vi "mobileye_paser.vi"() -> ()   [LabVIEW 2015]
uses:
  G_LCM.vi
  G_mobileye_Temp.vi
panel:
  out "mobileye time":u32=2087256306
  out "XY Graph":cluster{"Y":dbl[], "Y":dbl[]}[](graph)=[{"Y"=[1.82421875, 1.8301353427767753, 1.835194070339203, 1.8394013252854347, 1.8427635002136231, 1.84528698772192, 1.8469781804084777, 1.8478434708714486, 1.8478892517089844, 1.8471219155192375, 1.84554785490036, 1.8431734624505043, 1.8400051307678222, 1.8360492524504661, 1.8313122200965881, 1.8258004263043404, 1.819520263671875, 1.8124781247973443, 1.8046804022789003, 1.796133488714695, 1.7868437767028809, 1.77681765884161, 1.7660615277290344, 1.7545817759633064, 1.742384796142578, 1.7294769808650017, 1.7158647227287291, 1.701554414331913, 1.686552448272705, 1.6708652171492577, 1.654499113559723, 1.637460530102253, 1.619755859375, 1.6013914939761162, 1.5823738265037537, 1.5627092495560646, 1.5424041557312012, 1.5214649376273155, 1.4998979878425598, 1.4777096989750862, 1.4549064636230469, 1.431494674384594, 1.4074807238578795, 1.3828710046410562, 1.3576719093322753, 1.3318898305296898, 1.3055311608314515, 1.2786022928357124, 1.251109619140625, 1.2230595323443412], "Y"=[0.0, 0.5, 1.0, 1.5, 2.0, 2.5, 3.0, 3.5, 4.0, 4.5, 5.0, 5.5, 6.0, 6.5, 7.0, 7.5, 8.0, 8.5, 9.0, 9.5, 10.0, 10.5, 11.0, 11.5, 12.0, 12.5, 13.0, 13.5, 14.0, 14.5, 15.0, 15.5, 16.0, 16.5, 17.0, 17.5, 18.0, 18.5, 19.0, 19.5, 20.0, 20.5, 21.0, 21.5, 22.0, 22.5, 23.0, 23.5, 24.0, 24.5]}, {"Y"=[-1.22265625, -1.2167396572232247, -1.211680929660797, -1.2074736747145653, -1.2041114997863769, -1.20158801227808, -1.1998968195915223, -1.1990315291285514, -1.1989857482910156, -1.1997530844807625, -1.20132714509964, -1.2037015375494957, -1.2068698692321778, -1.2108257475495339, -1.2155627799034119, -1.2210745736956596, -1.227354736328125, -1.2343968752026557, -1.2421945977210997, -1.250741511285305, -1.2600312232971191, -1.27005734115839, -1.2808134722709656, -1.2922932240366936, -1.304490203857422, -1.3173980191349983, -1.3310102772712709, -1.345320585668087, -1.360322551727295, -1.3760097828507423, -1.392375886440277, -1.409414469897747, -1.427119140625, -1.4454835060238838, -1.4645011734962463, -1.4841657504439354, -1.5044708442687988, -1.5254100623726845, -1.5469770121574402, -1.5691653010249138, -1.5919685363769531, -1.615380325615406, -1.6393942761421205, -1.6640039953589438, -1.6892030906677247, -1.7149851694703102, -1.7413438391685485, -1.7682727071642876, -1.795765380859375, -1.8238154676556588, -1.8524165749549866, -1.8815623101592065, -1.911246280670166, -1.9414620938897134, -1.972203357219696, -2.003463678061962, -2.0352366638183597, -2.0675159218907355, -2.1002950596809384, -2.1335676845908162, -2.167327404022217, -2.2015678253769875, -2.2362825560569766, -2.2714652034640315, -2.307109375, -2.3432086780667305, -2.3797567200660703, -2.4167471083998677, -2.4541734504699706, -2.4920293536782263, -2.530308425426483, -2.5690042731165885, -2.6081105041503907, -2.647620725929737, -2.687528545856476, -2.7278275713324547, -2.7685114097595216, -2.809573668539524, -2.8510079550743104, -2.892807876765728, -2.934967041015625, -2.977479055225849, -3.020337526798248, -3.0635360631346704, -3.107068271636963, -3.150927759706974, -3.1951081347465515, -3.2396030041575434, -3.284405975341797, -3.3295106557011604, -3.3749106526374817, -3.4205995735526087, -3.466571025848389, -3.51281861692667, -3.5593359541893004], "Y"=[0.0, 0.5, 1.0, 1.5, 2.0, 2.5, 3.0, 3.5, 4.0, 4.5, 5.0, 5.5, 6.0, 6.5, 7.0, 7.5, 8.0, 8.5, 9.0, 9.5, 10.0, 10.5, 11.0, 11.5, 12.0, 12.5, 13.0, 13.5, 14.0, 14.5, 15.0, 15.5, 16.0, 16.5, 17.0, 17.5, 18.0, 18.5, 19.0, 19.5, 20.0, 20.5, 21.0, 21.5, 22.0, 22.5, 23.0, 23.5, 24.0, 24.5, 25.0, 25.5, 26.0, 26.5, 27.0, 27.5, 28.0, 28.5, 29.0, 29.5, 30.0, 30.5, 31.0, 31.5, 32.0, 32.5, 33.0, 33.5, 34.0, 34.5, 35.0, 35.5, 36.0, 36.5, 37.0, 37.5, 38.0, 38.5, 39.0, 39.5, 40.0, 40.5, 41.0, 41.5, 42.0, 42.5, 43.0, 43.5, 44.0, 44.5, 45.0, 45.5, 46.0, 46.5, 47.0]}, {"Y"=[-0.94, 0.94, 0.94, -0.94, -0.94], "Y"=[-3.2, -3.2, 1.5, 1.5, -3.2]}, {"Y"=[1.984375, 1.978057861328125, 1.9718017578125, 1.965606689453125, 1.95947265625], "Y"=[0.0, 0.5, 1.0, 1.5, 2.0]}, {"Y"=[-5.28125, -5.267578125, -5.25390625, -5.240234375, -5.2265625], "Y"=[0.0, 0.5, 1.0, 1.5, 2.0]}]
  out "x_view":dbl[](array[numeric])=[0.0, 0.5, 1.0, 1.5, 2.0, 2.5, 3.0, 3.5, 4.0, 4.5, 5.0, 5.5, 6.0, 6.5, 7.0, 7.5, 8.0, 8.5, 9.0, 9.5, 10.0, 10.5, 11.0, 11.5, 12.0, 12.5, 13.0, 13.5, 14.0, 14.5, 15.0, 15.5, 16.0, 16.5, 17.0, 17.5, 18.0, 18.5, 19.0, 19.5, 20.0, 20.5, 21.0, 21.5, 22.0, 22.5, 23.0, 23.5, 24.0, 24.5, 25.0, 25.5, 26.0, 26.5, 27.0, 27.5, 28.0, 28.5, 29.0, 29.5, 30.0, 30.5, 31.0, 31.5, 32.0, 32.5, 33.0, 33.5, 34.0, 34.5, 35.0, 35.5, 36.0, 36.5, 37.0, 37.5, 38.0, 38.5, 39.0, 39.5, 40.0, 40.5, 41.0, 41.5, 42.0, 42.5, 43.0, 43.5, 44.0, 44.5, 45.0, 45.5, 46.0, 46.5, 47.0, 47.5, 48.0, 48.5, 49.0, 49.5, 50.0, 50.5, 51.0, 51.5, 52.0, 52.5, 53.0, 53.5, 54.0, 54.5, 55.0, 55.5, 56.0, 56.5, 57.0, 57.5, 58.0, 58.5, 59.0, 59.5, 60.0, 60.5, 61.0, 61.5, 62.0, 62.5, 63.0, 63.5, 64.0, 64.5, 65.0, 65.5, 66.0, 66.5, 67.0, 67.5, 68.0, 68.5, 69.0, 69.5, 70.0, 70.5, 71.0, 71.5, 72.0, 72.5, 73.0, 73.5, 74.0, 74.5, 75.0, 75.5, 76.0, 76.5, 77.0, 77.5, 78.0, 78.5, 79.0, 79.5, 80.0, 80.5, 81.0, 81.5, 82.0, 82.5, 83.0, 83.5, 84.0, 84.5, 85.0, 85.5, 86.0, 86.5, 87.0, 87.5, 88.0, 88.5, 89.0, 89.5, 90.0, 90.5, 91.0, 91.5, 92.0, 92.5, 93.0, 93.5, 94.0, 94.5, 95.0, 95.5, 96.0, 96.5, 97.0, 97.5, 98.0, 98.5, 99.0, 99.5, 100.0, 100.5, 101.0, 101.5, 102.0, 102.5, 103.0, 103.5, 104.0, 104.5, 105.0, 105.5, 106.0, 106.5, 107.0, 107.5, 108.0, 108.5, 109.0, 109.5, 110.0, 110.5, 111.0, 111.5, 112.0, 112.5, 113.0, 113.5, 114.0, 114.5, 115.0, 115.5, 116.0, 116.5, 117.0, 117.5, 118.0, 118.5, 119.0, 119.5, 120.0, 120.5, 121.0, 121.5, 122.0, 122.5, 123.0, 123.5, 124.0, 124.5, 125.0, 125.5, 126.0, 126.5, 127.0, 127.5, 128.0]
  out "M_STOP":bool
  out "M_vel_limit":dbl=70.0
  out "M_headway":dbl=inf
  out "next lane right":dbl[][](array[numeric])=[[2087253162.0, 2.0, 0.0, 3.0, 0.17, 1.984375, 0.0001220703125, 0.0, 2087254803.0, -0.0126953125, 0.0], [0.0, 0.0, 0.0, 0.0, 0.0, 0.0, 0.0, 0.0, 0.0, 0.0, 0.0], [0.0, 0.0, 0.0, 0.0, 0.0, 0.0, 0.0, 0.0, 0.0, 0.0, 0.0], [0.0, 0.0, 0.0, 0.0, 0.0, 0.0, 0.0, 0.0, 0.0, 0.0, 0.0]]
  out "next lane left":dbl[][](array[numeric])=[[2087249118.0, 2.0, 0.0, 3.0, 0.19, -5.28125, 0.0, 0.0, 2087250819.0, 0.02734375, 0.0], [0.0, 0.0, 0.0, 0.0, 0.0, 0.0, 0.0, 0.0, 0.0, 0.0, 0.0], [0.0, 0.0, 0.0, 0.0, 0.0, 0.0, 0.0, 0.0, 0.0, 0.0, 0.0], [0.0, 0.0, 0.0, 0.0, 0.0, 0.0, 0.0, 0.0, 0.0, 0.0, 0.0]]
  out "lane_right":dbl[](array[numeric])=[2087240169.0, 0.0, 2.0, 3.0, 0.18, 1.82421875, -0.001728515625, 8.52346420288086e-06, 2087241810.0, 0.0126953125, 25.046875]
  out "lane_left":dbl[](array[numeric])=[2087236146.0, 4.0, 2.0, 3.0, 0.18, -1.22265625, -0.001728515625, 8.52346420288086e-06, 2087237829.0, 0.0126953125, 47.96875]
  out "obs_tmp":dbl[][](array[numeric])=[[7.0, 29.0625, -3.75, 3.5625, 0.0, 3.0, 1.0, 0.0, 31.5, 1.55, 115.0, 2.0, 1.0, 125.59, -0.017, 5.64, 7.390000000000001, 362446576.0], [0.0, 0.0, 0.0, 0.0, 0.0, 0.0, 0.0, 0.0, 0.0, 0.0, 0.0, 0.0, 0.0, 0.0, 0.0, 0.0, 0.0, 0.0], [0.0, 0.0, 0.0, 0.0, 0.0, 0.0, 0.0, 0.0, 0.0, 0.0, 0.0, 0.0, 0.0, 0.0, 0.0, 0.0, 0.0, 0.0], [0.0, 0.0, 0.0, 0.0, 0.0, 0.0, 0.0, 0.0, 0.0, 0.0, 0.0, 0.0, 0.0, 0.0, 0.0, 0.0, 0.0, 0.0], [0.0, 0.0, 0.0, 0.0, 0.0, 0.0, 0.0, 0.0, 0.0, 0.0, 0.0, 0.0, 0.0, 0.0, 0.0, 0.0, 0.0, 0.0], [0.0, 0.0, 0.0, 0.0, 0.0, 0.0, 0.0, 0.0, 0.0, 0.0, 0.0, 0.0, 0.0, 0.0, 0.0, 0.0, 0.0, 0.0], [0.0, 0.0, 0.0, 0.0, 0.0, 0.0, 0.0, 0.0, 0.0, 0.0, 0.0, 0.0, 0.0, 0.0, 0.0, 0.0, 0.0, 0.0], [0.0, 0.0, 0.0, 0.0, 0.0, 0.0, 0.0, 0.0, 0.0, 0.0, 0.0, 0.0, 0.0, 0.0, 0.0, 0.0, 0.0, 0.0], [0.0, 0.0, 0.0, 0.0, 0.0, 0.0, 0.0, 0.0, 0.0, 0.0, 0.0, 0.0, 0.0, 0.0, 0.0, 0.0, 0.0, 0.0], [0.0, 0.0, 0.0, 0.0, 0.0, 0.0, 0.0, 0.0, 0.0, 0.0, 0.0, 0.0, 0.0, 0.0, 0.0, 0.0, 0.0, 0.0], [0.0, 0.0, 0.0, 0.0, 0.0, 0.0, 0.0, 0.0, 0.0, 0.0, 0.0, 0.0, 0.0, 0.0, 0.0, 0.0, 0.0, 0.0], [0.0, 0.0, 0.0, 0.0, 0.0, 0.0, 0.0, 0.0, 0.0, 0.0, 0.0, 0.0, 0.0, 0.0, 0.0, 0.0, 0.0, 0.0], [0.0, 0.0, 0.0, 0.0, 0.0, 0.0, 0.0, 0.0, 0.0, 0.0, 0.0, 0.0, 0.0, 0.0, 0.0, 0.0, 0.0, 0.0], [0.0, 74.9375, 0.0, 0.0, 0.0, 0.0, 0.0, 0.0, 0.0, 0.0, 0.0, 0.0, 0.0, 0.0, 0.0, 0.0, 0.0, 0.0], [0.0, 0.0, 0.0, 0.0, 0.0, 0.0, 0.0, 0.0, 0.0, 0.0, 0.0, 0.0, 0.0, 0.0, 0.0, 0.0, 0.0, 0.0], [0.0, 0.0, 0.0, 0.0, 0.0, 0.0, 0.0, 0.0, 0.0, 0.0, 0.0, 0.0, 0.0, 0.0, 0.0, 0.0, 0.0, 0.0], [0.0, 0.0, 0.0, 0.0, 0.0, 0.0, 0.0, 0.0, 0.0, 0.0, 0.0, 0.0, 0.0, 0.0, 0.0, 0.0, 0.0, 0.0], [0.0, 0.0, 0.0, 0.0, 0.0, 0.0, 0.0, 0.0, 0.0, 0.0, 0.0, 0.0, 0.0, 0.0, 0.0, 0.0, 0.0, 0.0], [0.0, 0.0, 0.0, 0.0, 0.0, 0.0, 0.0, 0.0, 0.0, 0.0, 0.0, 0.0, 0.0, 0.0, 0.0, 0.0, 0.0, 0.0], [0.0, 0.0, 0.0, 0.0, 0.0, 0.0, 0.0, 0.0, 0.0, 0.0, 0.0, 0.0, 0.0, 0.0, 0.0, 0.0, 0.0, 0.0], [0.0, 0.0, 0.0, 0.0, 0.0, 0.0, 0.0, 0.0, 0.0, 0.0, 0.0, 0.0, 0.0, 0.0, 0.0, 0.0, 0.0, 0.0], [0.0, 0.0, 0.0, 0.0, 0.0, 0.0, 0.0, 0.0, 0.0, 0.0, 0.0, 0.0, 0.0, 0.0, 0.0, 0.0, 0.0, 0.0], [0.0, 0.0, 0.0, 0.0, 0.0, 0.0, 0.0, 0.0, 0.0, 0.0, 0.0, 0.0, 0.0, 0.0, 0.0, 0.0, 0.0, 0.0], [0.0, 0.0, 0.0, 0.0, 0.0, 0.0, 0.0, 0.0, 0.0, 0.0, 0.0, 0.0, 0.0, 0.0, 0.0, 0.0, 0.0, 0.0], [0.0, 0.0, 0.0, 0.0, 0.0, 0.0, 0.0, 0.0, 0.0, 0.0, 0.0, 0.0, 0.0, 0.0, 0.0, 0.0, 0.0, 0.0], [0.0, 0.0, 0.0, 0.0, 0.0, 0.0, 0.0, 0.0, 0.0, 0.0, 0.0, 0.0, 0.0, 0.0, 0.0, 0.0, 0.0, 0.0], [0.0, 0.0, 0.0, 0.0, 0.0, 0.0, 0.0, 0.0, 0.0, 0.0, 0.0, 0.0, 0.0, 0.0, 0.0, 0.0, 0.0, 0.0], [0.0, 0.0, 0.0, 0.0, 0.0, 0.0, 0.0, 0.0, 0.0, 0.0, 0.0, 0.0, 0.0, 0.0, 0.0, 0.0, 0.0, 0.0], [0.0, 0.0, 0.0, 0.0, 0.0, 0.0, 0.0, 0.0, 0.0, 0.0, 0.0, 0.0, 0.0, 0.0, 0.0, 0.0, 0.0, 0.0], [0.0, 0.0, 0.0, 0.0, 0.0, 0.0, 0.0, 0.0, 0.0, 0.0, 0.0, 0.0, 0.0, 0.0, 0.0, 0.0, 0.0, 0.0], [0.0, 0.0, 0.0, 0.0, 0.0, 0.0, 0.0, 0.0, 0.0, 0.0, 0.0, 0.0, 0.0, 0.0, 0.0, 0.0, 0.0, 0.0], [0.0, 0.0, 0.0, 0.0, 0.0, 0.0, 0.0, 0.0, 0.0, 0.0, 0.0, 0.0, 0.0, 0.0, 0.0, 0.0, 0.0, 0.0], [0.0, 0.0, 0.0, 0.0, 0.0, 0.0, 0.0, 0.0, 0.0, 0.0, 0.0, 0.0, 0.0, 0.0, 0.0, 0.0, 0.0, 0.0], [0.0, 0.0, 0.0, 0.0, 0.0, 0.0, 0.0, 0.0, 0.0, 0.0, 0.0, 0.0, 0.0, 0.0, 0.0, 0.0, 0.0, 0.0], [0.0, 0.0, 0.0, 0.0, 0.0, 0.0, 0.0, 0.0, 0.0, 0.0, 0.0, 0.0, 0.0, 0.0, 0.0, 0.0, 0.0, 0.0], [0.0, 0.0, 0.0, 0.0, 0.0, 0.0, 0.0, 0.0, 0.0, 0.0, 0.0, 0.0, 0.0, 0.0, 0.0, 0.0, 0.0, 0.0], [0.0, 0.0, 0.0, 0.0, 0.0, 0.0, 0.0, 0.0, 0.0, 0.0, 0.0, 0.0, 0.0, 0.0, 0.0, 0.0, 0.0, 0.0], [0.0, 0.0, 0.0, 0.0, 0.0, 0.0, 0.0, 0.0, 0.0, 0.0, 0.0, 0.0, 0.0, 0.0, 0.0, 0.0, 0.0, 0.0], [0.0, 0.0, 0.0, 0.0, 0.0, 0.0, 0.0, 0.0, 0.0, 0.0, 0.0, 0.0, 0.0, 0.0, 0.0, 0.0, 0.0, 0.0], [0.0, 0.0, 0.0, 0.0, 0.0, 0.0, 0.0, 0.0, 0.0, 0.0, 0.0, 0.0, 0.0, 0.0, 0.0, 0.0, 0.0, 0.0], [0.0, 0.0, 0.0, 0.0, 0.0, 0.0, 0.0, 0.0, 0.0, 0.0, 0.0, 0.0, 0.0, 0.0, 0.0, 0.0, 0.0, 0.0], [0.0, 0.0, 0.0, 0.0, 0.0, 0.0, 0.0, 0.0, 0.0, 0.0, 0.0, 0.0, 0.0, 0.0, 0.0, 0.0, 0.0, 0.0], [0.0, 0.0, 0.0, 0.0, 0.0, 0.0, 0.0, 0.0, 0.0, 0.0, 0.0, 0.0, 0.0, 0.0, 0.0, 0.0, 0.0, 0.0], [0.0, 0.0, 0.0, 0.0, 0.0, 0.0, 0.0, 0.0, 0.0, 0.0, 0.0, 0.0, 0.0, 0.0, 0.0, 0.0, 0.0, 0.0], [0.0, 0.0, 0.0, 0.0, 0.0, 0.0, 0.0, 0.0, 0.0, 0.0, 0.0, 0.0, 0.0, 0.0, 0.0, 0.0, 0.0, 0.0], [0.0, 0.0, 0.0, 0.0, 0.0, 0.0, 0.0, 0.0, 0.0, 0.0, 0.0, 0.0, 0.0, 0.0, 0.0, 0.0, 0.0, 0.0], [0.0, 0.0, 0.0, 0.0, 0.0, 0.0, 0.0, 0.0, 0.0, 0.0, 0.0, 0.0, 0.0, 0.0, 0.0, 0.0, 0.0, 0.0], [0.0, 0.0, 0.0, 0.0, 0.0, 0.0, 0.0, 0.0, 0.0, 0.0, 0.0, 0.0, 0.0, 0.0, 0.0, 0.0, 0.0, 0.0], [0.0, 0.0, 0.0, 0.0, 0.0, 0.0, 0.0, 0.0, 0.0, 0.0, 0.0, 0.0, 0.0, 0.0, 0.0, 0.0, 0.0, 0.0], [0.0, 0.0, 0.0, 0.0, 0.0, 0.0, 0.0, 0.0, 0.0, 0.0, 0.0, 0.0, 0.0, 0.0, 0.0, 0.0, 0.0, 0.0], [0.0, 0.0, 0.0, 0.0, 0.0, 0.0, 0.0, 0.0, 0.0, 0.0, 0.0, 0.0, 0.0, 0.0, 0.0, 0.0, 0.0, 0.0], [0.0, 0.0, 0.0, 0.0, 0.0, 0.0, 0.0, 0.0, 0.0, 0.0, 0.0, 0.0, 0.0, 0.0, 0.0, 0.0, 0.0, 0.0], [0.0, 0.0, 0.0, 0.0, 0.0, 0.0, 0.0, 0.0, 0.0, 0.0, 0.0, 0.0, 0.0, 0.0, 0.0, 0.0, 0.0, 0.0], [0.0, 0.0, 0.0, 0.0, 0.0, 0.0, 0.0, 0.0, 0.0, 0.0, 0.0, 0.0, 0.0, 0.0, 0.0, 0.0, 0.0, 0.0], [0.0, 0.0, 0.0, 0.0, 0.0, 0.0, 0.0, 0.0, 0.0, 0.0, 0.0, 0.0, 0.0, 0.0, 0.0, 0.0, 0.0, 0.0], [0.0, 0.0, 0.0, 0.0, 0.0, 0.0, 0.0, 0.0, 0.0, 0.0, 0.0, 0.0, 0.0, 0.0, 0.0, 0.0, 0.0, 0.0], [0.0, 0.0, 0.0, 0.0, 0.0, 0.0, 0.0, 0.0, 0.0, 0.0, 0.0, 0.0, 0.0, 0.0, 0.0, 0.0, 0.0, 0.0], [0.0, 0.0, 0.0, 0.0, 0.0, 0.0, 0.0, 0.0, 0.0, 0.0, 0.0, 0.0, 0.0, 0.0, 0.0, 0.0, 0.0, 0.0], [0.0, 0.0, 0.0, 0.0, 0.0, 0.0, 0.0, 0.0, 0.0, 0.0, 0.0, 0.0, 0.0, 0.0, 0.0, 0.0, 0.0, 0.0], [0.0, 0.0, 0.0, 0.0, 0.0, 0.0, 0.0, 0.0, 0.0, 0.0, 0.0, 0.0, 0.0, 0.0, 0.0, 0.0, 0.0, 0.0], [0.0, 0.0, 0.0, 0.0, 0.0, 0.0, 0.0, 0.0, 0.0, 0.0, 0.0, 0.0, 0.0, 0.0, 0.0, 0.0, 0.0, 0.0], [0.0, 0.0, 0.0, 0.0, 0.0, 0.0, 0.0, 0.0, 0.0, 0.0, 0.0, 0.0, 0.0, 0.0, 0.0, 0.0, 0.0, 0.0], [0.0, 0.0, 0.0, 0.0, 0.0, 0.0, 0.0, 0.0, 0.0, 0.0, 0.0, 0.0, 0.0, 0.0, 0.0, 0.0, 0.0, 0.0], [0.0, 0.0, 0.0, 0.0, 0.0, 0.0, 0.0, 0.0, 0.0, 0.0, 0.0, 0.0, 0.0, 0.0, 0.0, 0.0, 0.0, 0.0]]
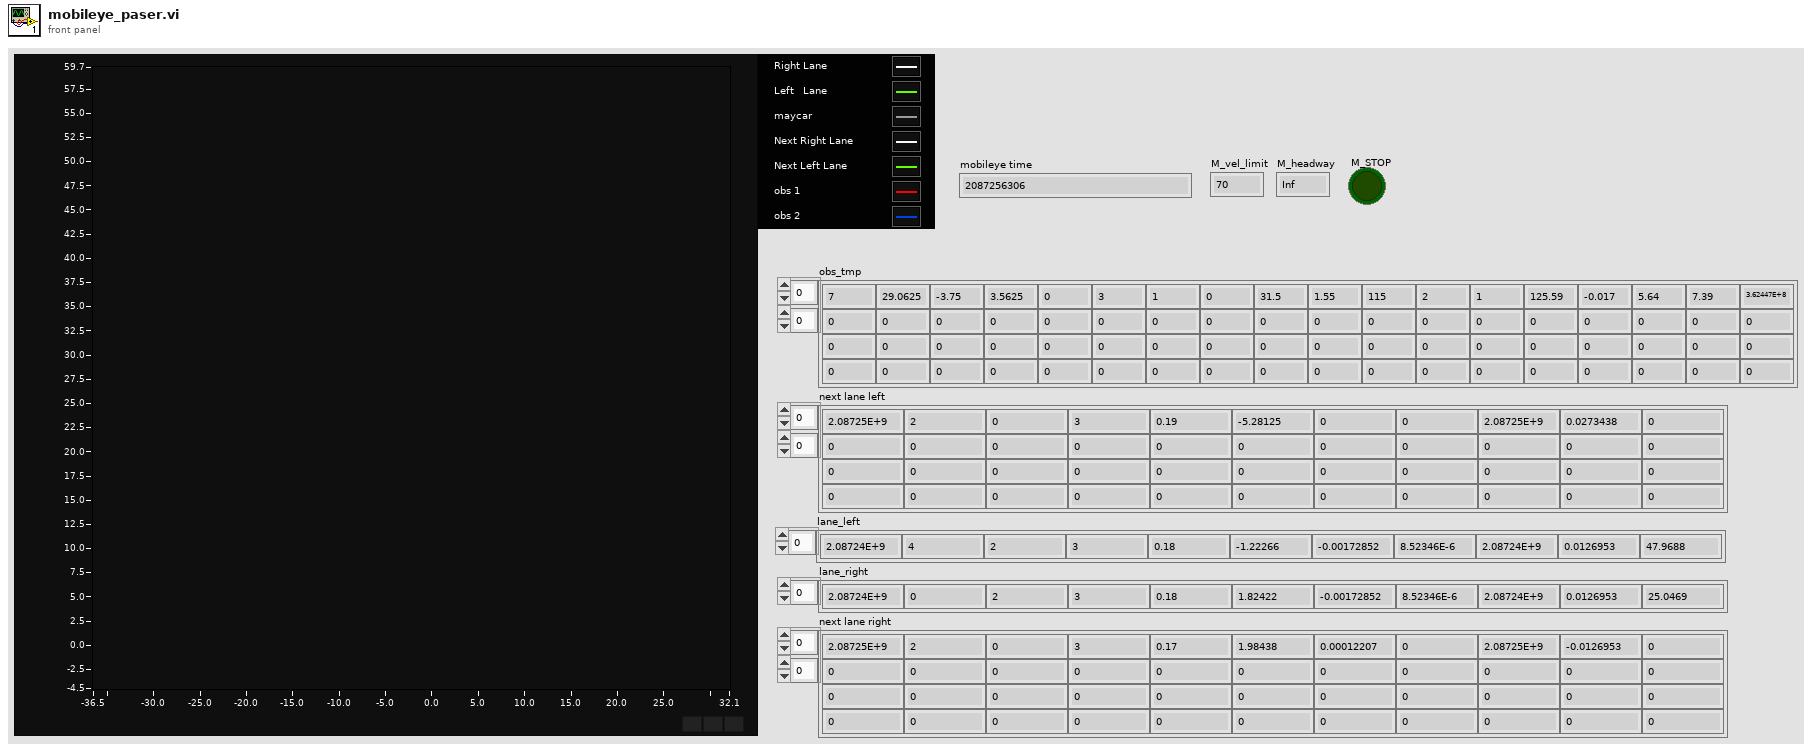
[diagram p1: front panel]
types:
  T1 = cluster{"hash":i64, "sys time":i64, "mobileye time":u32, "ID":u32, "data":u8[]}
  T2 = cluster{"identifier":u32, "timestamp":timestamp, "payload":u8[]}
  T3 = cluster{"hash":i64, "sys time":i64, "car time":u32, "ID":u32, "data":u8[]}
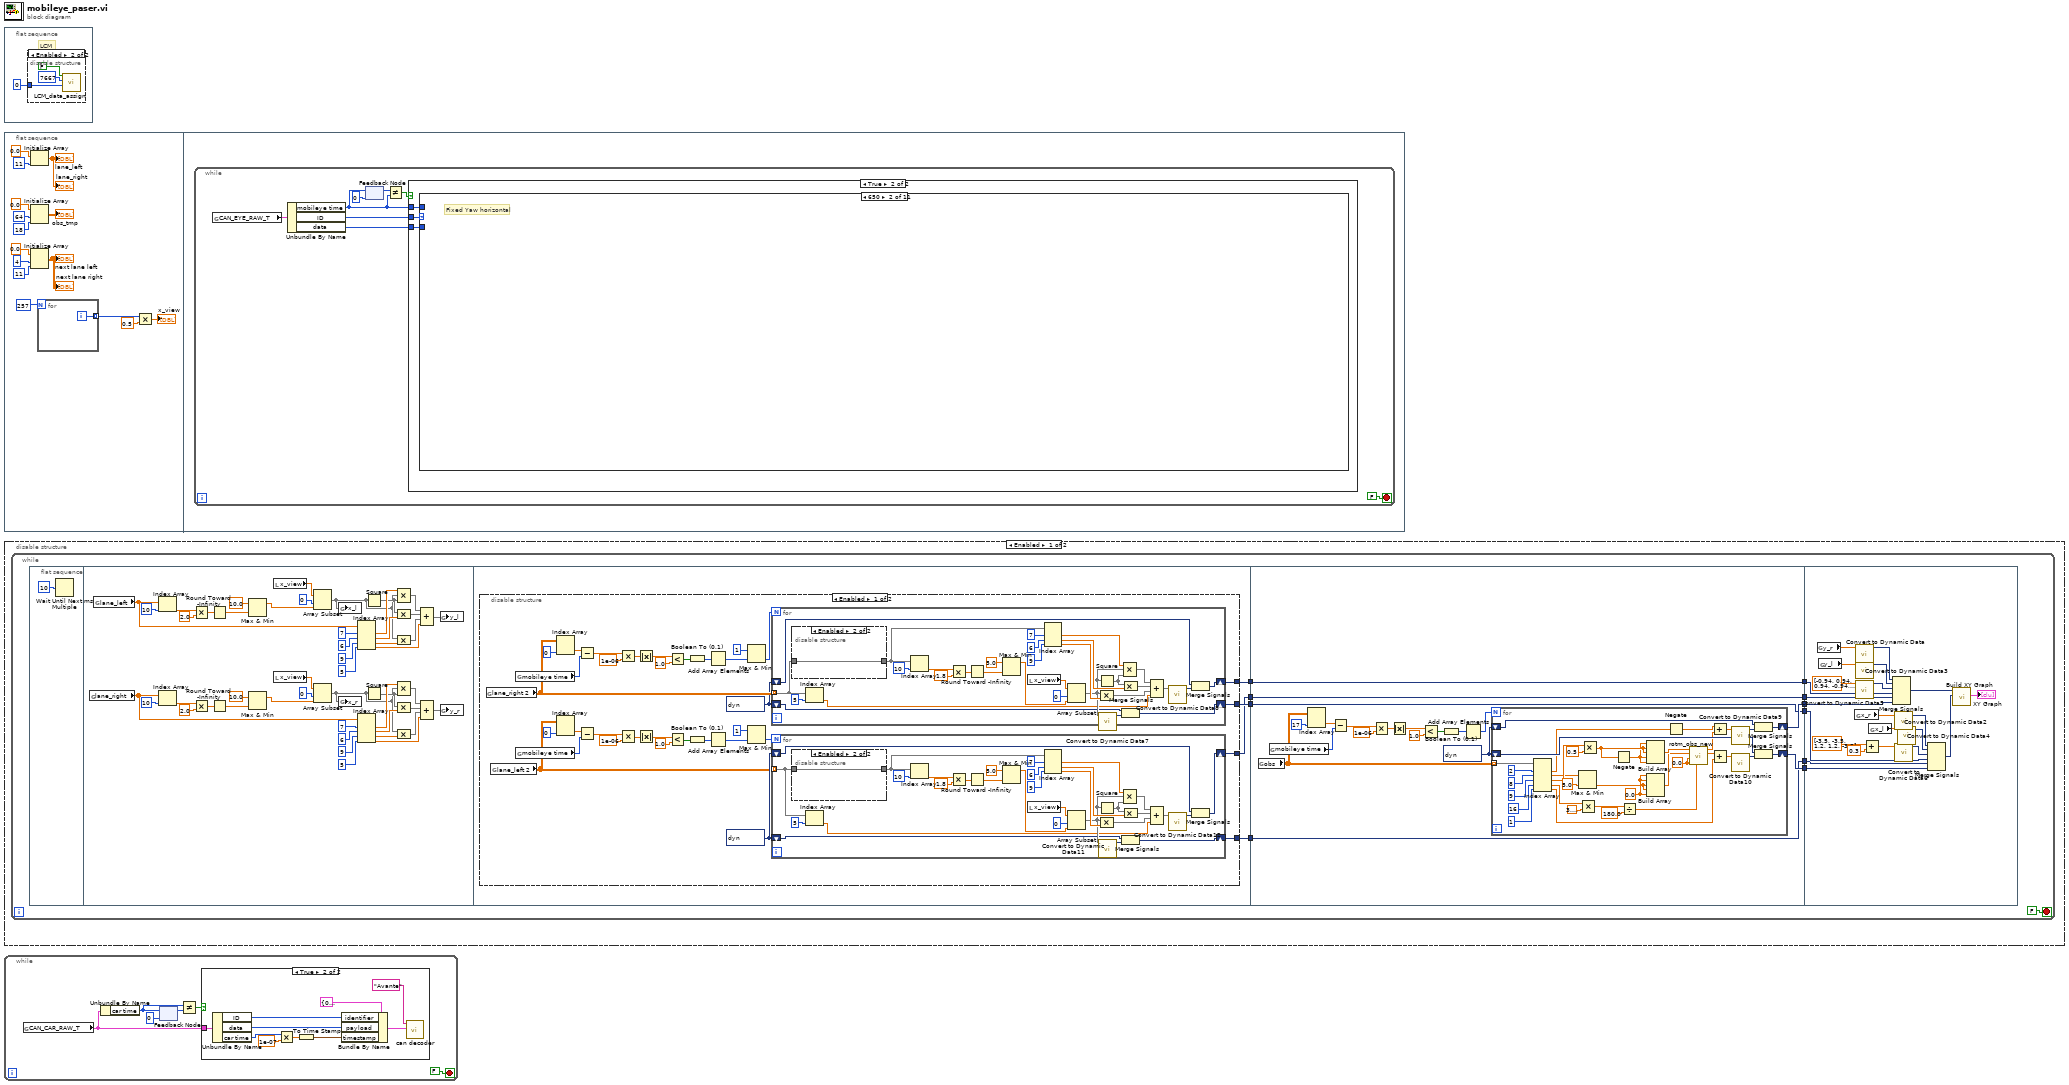
[diagram p0: block diagram]
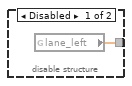
[diagram p3: hidden frame]
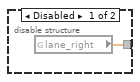
[diagram p4: hidden frame]
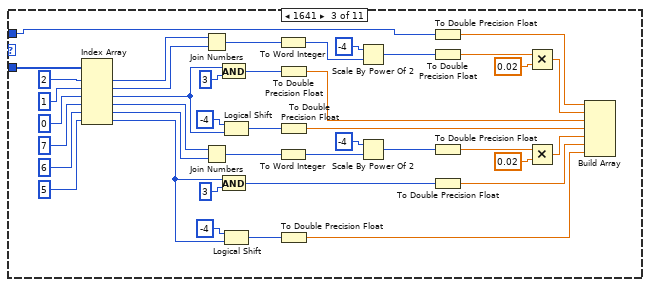
[diagram p9: hidden frame]
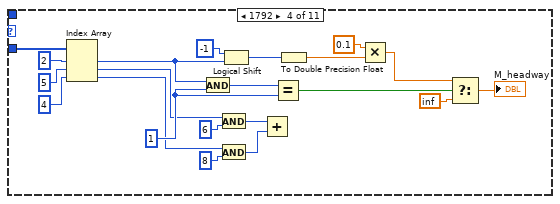
[diagram p10: hidden frame]
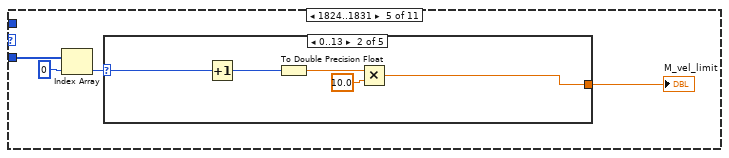
[diagram p11: hidden frame]
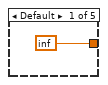
[diagram p12: hidden frame]
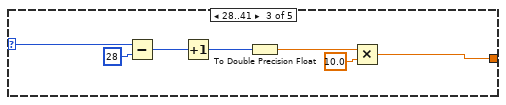
[diagram p13: hidden frame]
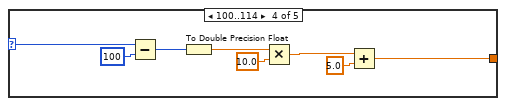
[diagram p14: hidden frame]
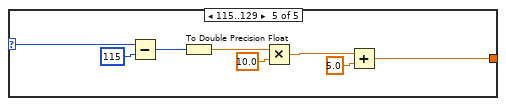
[diagram p15: hidden frame]
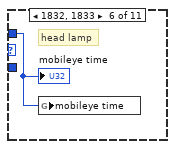
[diagram p16: hidden frame]
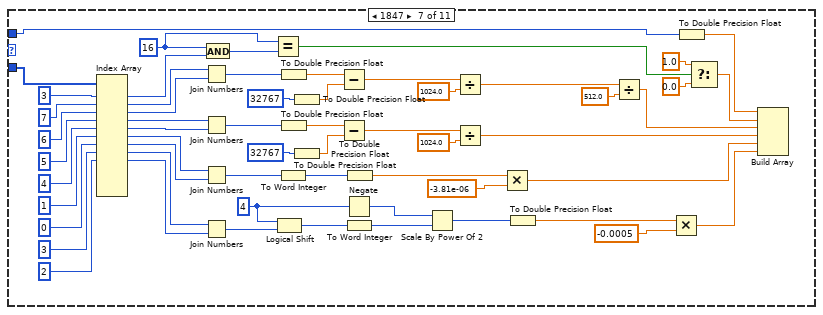
[diagram p17: hidden frame]
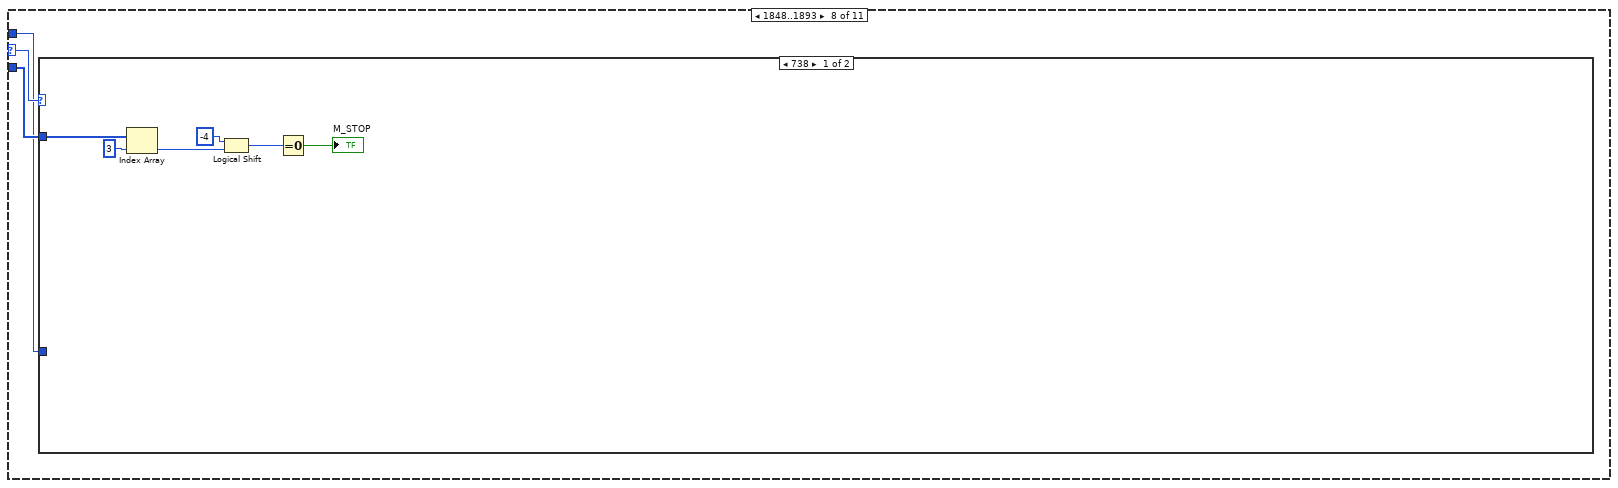
[diagram p18: hidden frame]
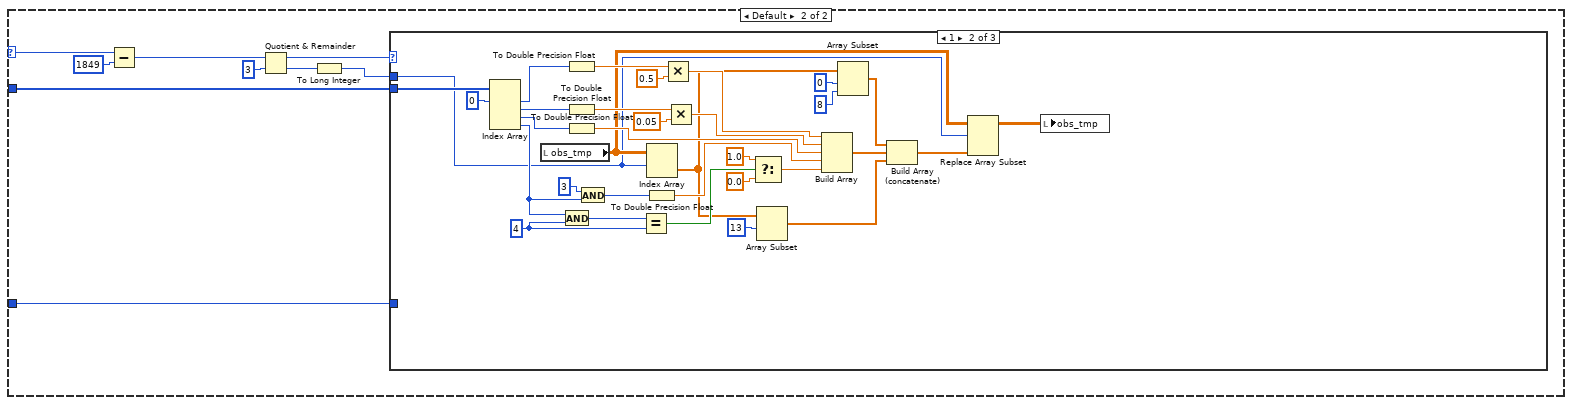
[diagram p19: hidden frame]
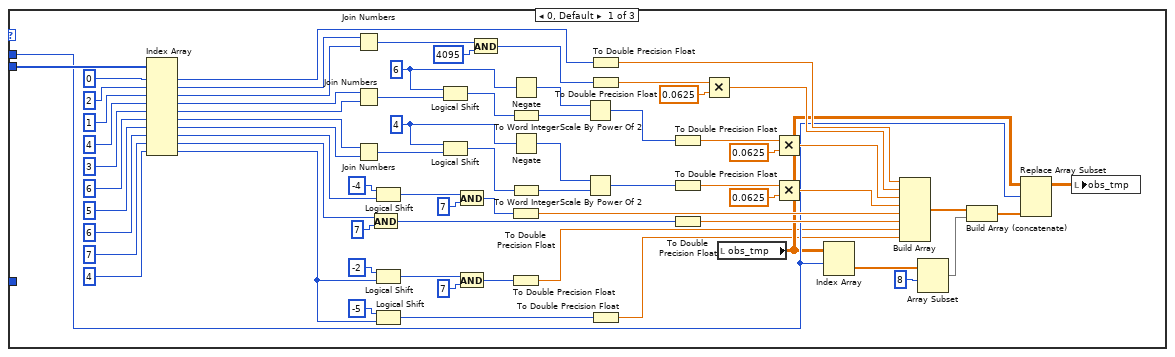
[diagram p20: hidden frame]
diagram:
  n1 = flat-sequence {
    frame #0 {
      # "LCM"
      n2 = disable-structure shown="Enabled" {
        disable-tunnel: u16 0 ("time-to-live") -> [_ w2]
        frame Disabled {
          n3 = call "comm.vi"() -> ()  [unwired: 12 in]
        }
        frame Enabled {
          n4 = call "LCM_data_assign.vi"("time-to-live"=w2, "port"=u16 7667, "velodyne enable"=FALSE) -> ()  [unwired: 9 in]
        }
      }
    }
  }
  n5 = flat-sequence {
    frame #0 {
      n6 = Initialize Array(0.0, 11 ("dimension size")) -> (→"lane_left" →"lane_right":dbl[])
      n7 = Initialize Array(0.0 ("element"), 64 ("dimension size"), 18 ("dimension size")) -> (→"obs_tmp":dbl[][])
      n8 = Initialize Array(0.0, 4 ("dimension size"), 11 ("dimension size")) -> (→"next lane right" →"next lane left":dbl[][])
      n9 = for {
        N: 257 -> [_]
        tunnel: [w20] -> w11 mode=indexing
        i -> [w20]
      }
      n10 = Multiply(x=w11, y=0.5) -> (x*y=→"x_view":dbl[])
    }
    frame #1 {
      n11 = while {
        stop <- FALSE stop-if-true
        n12 = global read "G_LCM.vi" "CAN_EYE_RAW_T"() -> (w27:T1)
        n13 = Unbundle By Name(w27) -> ("mobileye time"=w22:u32, "ID"=w23:u32, "data"=w24:u8[])
        n14 = feedback #1(u32 0 ("mobileye time")) -> (w21:u32)
        n15 = feedback-in #1(w22) -> ()
        n16 = Not Equal?(x=w21, y=w22) -> (x != y?=w25:bool)
        n17 = case shown="True" w25 {
          tunnel: w24 -> [_ w31]
          tunnel: w22 -> [_ w30]
          tunnel: w23 -> [_ w29]
          frame False {
          }
          frame True {
            n18 = case shown="650" w29 {
              selector: w29 -> [_ _ _ _ _ _ _ w187 _ w393 w475]
              tunnel: w31 -> [_ _ w72 w93 w97 _ w184 w186 w362 w447 w502]
              tunnel: w30 -> [_ _ w49 _ _ w127 w131 w185 _ w413 w478]
              frame 0, Default {
              }
              frame 1616 {
                # "Fixed Yaw horizontal"
              }
              frame 1641 {
                n19 = Index Array(array=w72, index #1=2 ("index"), index #2=1 ("index"), index #3=0 ("index"), index #4=7 ("index"), index #5=6 ("index"), index #6=5 ("index")) -> (element #1=w69:u8, element #2=w68:u8, element #3=w47:u8, element #4=w40:u8, element #5=w39:u8, element #6=w35:u8)
                n20 = Join Numbers(hi=w69, lo=w68) -> ((hi.lo)=w67:u16)
                n21 = Join Numbers(hi=w40, lo=w39) -> ((hi.lo)=w62:u16)
                n22 = And(x=w47, y=u8 3) -> (x .and. y?=w46:u8)
                n23 = And(x=w35, y=u8 3) -> (x .and. y?=w38:u8)
                n24 = Logical Shift(y=i16 -4, x=w47) -> (x << y=w45:u8)
                n25 = Logical Shift(y=i16 -4, x=w35) -> (x << y=w42:u8)
                n26 = To Word Integer(number=w67) -> (16bit integer=w54:i16)
                n27 = To Word Integer(number=w62) -> (16bit integer=w51:i16)
                n28 = To Double Precision Float(number=w46) -> (double precision float=w44:dbl)
                n29 = To Double Precision Float(number=w45) -> (double precision float=w43:dbl)
                n30 = To Double Precision Float(number=w42) -> (double precision float=w36:dbl)
                n31 = Scale By Power Of 2(n=i16 -4 ("y"), x=w54) -> (x*2^n=w53:i16)
                n32 = Scale By Power Of 2(n=i16 -4 ("y"), x=w51) -> (x*2^n=w50:i16)
                n33 = To Double Precision Float(number=w49) -> (double precision float=w34:dbl)
                n34 = To Double Precision Float(number=w53) -> (double precision float=w66:dbl)
                n35 = To Double Precision Float(number=w50) -> (double precision float=w63:dbl)
                n36 = To Double Precision Float(number=w38) -> (double precision float=w37:dbl)
                n37 = Multiply(x=w66, y=0.02) -> (x*y=w33:dbl)
                n38 = Multiply(x=w63, y=0.02) -> (x*y=w32:dbl)
                n39 = Build Array(w34, w33, w44, w43, w32, w37, w36) -> ()  [unwired: 1 out]
              }
              frame 1792 {
                w88 = u8 1 ("y")
                n40 = Index Array(array=w93, index #1=2 ("index"), index #2=5 ("index"), index #3=4 ("index")) -> (element #1=w91:u8, element #2=w80:u8, element #3=w76:u8)
                n41 = And(x=w91, y=w88) -> (x .and. y?=w89:u8)
                n42 = And(x=w80, y=u8 6) -> (x .and. y?=w75:u8)
                n43 = And(x=w76, y=u8 8) -> (x .and. y?=w74:u8)
                n44 = Logical Shift(y=i16 -1, x=w91) -> (x << y=w86:u8)
                n45 = Add(x=w75, y=w74) -> ()  [unwired: 1 out]
                n46 = Equal?(x=w89, y=w88) -> (x = y?=w87:bool)
                n47 = To Double Precision Float(number=w86) -> (double precision float=w85:dbl)
                n48 = Multiply(x=0.1, y=w85) -> (x*y=w83:dbl)
                n49 = Select(t=w83, s=w87, f=inf) -> (s? t:f=→"M_headway":dbl)
              }
              frame 1824..1831 {
                n50 = Index Array(array=w97, index=0) -> (element=w95:u8)
                n51 = case shown="0..13" w95 {
                  selector: w95 -> [_ w103 w106 w116 w124]
                  tunnel: [inf w99 w107 w111 w119] -> w94
                  frame Default {
                  }
                  frame 0..13 {
                    n52 = Increment(x=w103) -> (x+1=w102:u8)
                    n53 = To Double Precision Float(number=w102) -> (double precision float=w101:dbl)
                    n54 = Multiply(x=w101, y=10.0) -> (x*y=w99:dbl)
                  }
                  frame 28..41 {
                    n55 = Subtract(x=w106, y=u8 28) -> (x-y=w105:u8)
                    n56 = Increment(x=w105) -> (x+1=w110:u8)
                    n57 = To Double Precision Float(number=w110) -> (double precision float=w109:dbl)
                    n58 = Multiply(x=w109, y=10.0) -> (x*y=w107:dbl)
                  }
                  frame 100..114 {
                    n59 = Subtract(x=w116, y=u8 100) -> (x-y=w114:u8)
                    n60 = To Double Precision Float(number=w114) -> (double precision float=w118:dbl)
                    n61 = Multiply(x=w118, y=10.0) -> (x*y=w113:dbl)
                    n62 = Add(x=w113, y=5.0) -> (x+y=w111:dbl)
                  }
                  frame 115..129 {
                    n63 = Subtract(x=w124, y=u8 115) -> (x-y=w122:u8)
                    n64 = To Double Precision Float(number=w122) -> (double precision float=w126:dbl)
                    n65 = Multiply(x=w126, y=10.0) -> (x*y=w121:dbl)
                    n66 = Add(x=w121, y=5.0) -> (x+y=w119:dbl)
                  }
                }
                "M_vel_limit" <- w94
              }
              frame 1832, 1833 {
                # "head lamp"
                n67 = global write "G_mobileye_Temp.vi" "mobileye time"(w127) -> ()
                "mobileye time" <- w127
              }
              frame 1847 {
                w164 = u8 16 ("x")
                w166 = i16 4 ("x")
                n68 = Index Array(array=w184, index #1=3 ("index"), index #2=7 ("index"), index #3=6 ("index"), index #4=5 ("index"), index #5=4 ("index"), index #6=1 ("index"), index #7=0 ("index"), index #8=3 ("index"), index #9=2 ("index")) -> (element #1=w147:u8, element #2=w141:u8, element #3=w140:u8, element #4=w139:u8, element #5=w138:u8, element #6=w181:u8, element #7=w180:u8, element #8=w173:u8, element #9=w172:u8)  [unwired: 4 in, 4 out]
                n69 = Join Numbers(hi=w141, lo=w140) -> ((hi.lo)=w163:u16)
                n70 = Join Numbers(hi=w139, lo=w138) -> ((hi.lo)=w151:u16)
                n71 = Join Numbers(hi=w181, lo=w180) -> ((hi.lo)=w179:u16)
                n72 = Join Numbers(hi=w173, lo=w172) -> ((hi.lo)=w169:u16)
                n73 = And(x=w164, y=w147) -> (x .and. y?=w165:u8)
                n74 = Equal?(x=w164, y=w165) -> (x = y?=w150:bool)
                n75 = Logical Shift(y=w166, x=w169) -> (x << y=w171:u16)
                n76 = To Word Integer(number=w179) -> (16bit integer=w178:i16)
                n77 = To Double Precision Float(number=w163) -> (double precision float=w162:dbl)
                n78 = To Double Precision Float(number=w151) -> (double precision float=w152:dbl)
                n79 = To Double Precision Float(number=i16 32767) -> (double precision float=w160:dbl)
                n80 = To Double Precision Float(number=i16 32767) -> (double precision float=w154:dbl)
                n81 = Subtract(x=w162, y=w160) -> (x-y=w159:dbl)
                n82 = Subtract(x=w152, y=w154) -> (x-y=w155:dbl)
                n83 = Negate(x=w166) -> (-x=w168:i16)
                n84 = To Word Integer(number=w171) -> (16bit integer=w128:i16)
                n85 = To Double Precision Float(number=w178) -> (double precision float=w177:dbl)
                n86 = Scale By Power Of 2(n=w168, x=w128) -> (x*2^n=w167:i16)
                n87 = Divide(x=w159, y=1024.0) -> (x/y=w136:dbl)
                n88 = Divide(x=w155, y=1024.0) -> (x/y=w134:dbl)
                n89 = Multiply(x=w177, y=-3.81e-06) -> (x*y=w133:dbl)
                n90 = To Double Precision Float(number=w167) -> (double precision float=w129:dbl)
                n91 = Divide(x=w136, y=512.0) -> (x/y=w135:dbl)
                n92 = Multiply(x=w129, y=-0.0005) -> (x*y=w132:dbl)
                n93 = To Double Precision Float(number=w131) -> (double precision float=w130:dbl)
                n94 = Select(t=1.0, s=w150, f=0.0) -> (s? t:f=w137:dbl)
                n95 = Build Array(w130, w137, w135, w134, w133, w132) -> ()  [unwired: 1 out]
              }
              frame 1848..1893 {
                n96 = case shown="738" w187 {
                  selector: w187 -> [_ w196]
                  tunnel: w186 -> [w193 w198]
                  tunnel: w185 -> [_ w194]
                  frame 1848 {
                    n97 = Index Array(array=w193, index=3) -> (element=w189:u8)
                    n98 = Logical Shift(y=i16 -4, x=w189) -> (x << y=w191:u8)
                    n99 = Equal To 0?(x=w191) -> (x = 0?=→"M_STOP":bool)
                  }
                  frame Default {
                    n100 = Subtract(x=w196, y=u32 1849) -> (x-y=w201:u32)
                    n101 = Quotient & Remainder(x=w201, y=u32 3) -> (x-y*floor(x/y)=w199:u32, floor(x/y)=w197:u32)
                    n102 = To Long Integer(number=w197) -> (32bit integer=w195:i32)
                    n103 = case shown="1" w199 {
                      tunnel: w198 -> [w272 w305 w308]
                      tunnel: w195 -> [w226 w280 w307]
                      tunnel: w194 -> [_ _ w306]
                      frame 0, Default {
                        w215 = i16 4 ("y")
                        w219 = i16 6 ("y")
                        n104 = Index Array(array=w272, index #1=0 ("index"), index #2=2 ("index"), index #3=1 ("index"), index #4=4 ("index"), index #5=3 ("index"), index #6=6 ("index"), index #7=5 ("index"), index #8=6 ("index"), index #9=7 ("index"), index #10=4 ("index")) -> (element #1=w264:u8, element #2=w268:u8, element #3=w267:u8, element #4=w256:u8, element #5=w255:u8, element #6=w243:u8, element #7=w242:u8, element #8=w238:u8, element #9=w231:u8, element #10=w206:u8)
                        n105 = Join Numbers(hi=w268, lo=w267) -> ((hi.lo)=w259:u16)
                        n106 = Join Numbers(hi=w256, lo=w255) -> ((hi.lo)=w254:u16)
                        n107 = Join Numbers(hi=w243, lo=w242) -> ((hi.lo)=w244:u16)
                        n108 = And(x=w231, y=u8 7) -> (x .and. y?=w230:u8)
                        n109 = Logical Shift(y=i16 -4, x=w238) -> (x << y=w237:u8)
                        n110 = Logical Shift(y=i16 -2, x=w206) -> (x << y=w210:u8)
                        n111 = Logical Shift(y=i16 -5, x=w206) -> (x << y=w204:u8)
                        n112 = Logical Shift(y=w219, x=w254) -> (x << y=w253:u16)
                        n113 = Logical Shift(y=w215, x=w244) -> (x << y=w245:u16)
                        n114 = And(x=w237, y=u8 7) -> (x .and. y?=w235:u8)
                        n115 = And(x=w210, y=u8 7) -> (x .and. y?=w208:u8)
                        n116 = And(x=w259, y=u16 4095) -> (x .and. y?=w265:u16)
                        n117 = Negate(x=w219) -> (-x=w220:i16)
                        n118 = To Word Integer(number=w253) -> (16bit integer=w218:i16)
                        n119 = Negate(x=w215) -> (-x=w216:i16)
                        n120 = To Word Integer(number=w245) -> (16bit integer=w214:i16)
                        n121 = To Double Precision Float(number=w235) -> (double precision float=w234:dbl)
                        n122 = To Double Precision Float(number=w208) -> (double precision float=w207:dbl)
                        n123 = Scale By Power Of 2(n=w220, x=w218) -> (x*2^n=w217:i16)
                        n124 = Scale By Power Of 2(n=w216, x=w214) -> (x*2^n=w213:i16)
                        n125 = To Double Precision Float(number=w264) -> (double precision float=w261:dbl)
                        n126 = To Double Precision Float(number=w265) -> (double precision float=w263:dbl)
                        n127 = To Double Precision Float(number=w204) -> (double precision float=w203:dbl)
                        n128 = To Double Precision Float(number=w217) -> (double precision float=w250:dbl)
                        n129 = To Double Precision Float(number=w213) -> (double precision float=w247:dbl)
                        n130 = To Double Precision Float(number=w230) -> (double precision float=w229:dbl)
                        n131 = Multiply(x=w263, y=0.0625) -> (x*y=w260:dbl)
                        n132 = local read "obs_tmp"() -> (w225:dbl[][])
                        n133 = Multiply(x=w250, y=0.0625) -> (x*y=w251:dbl)
                        n134 = Multiply(x=w247, y=0.0625) -> (x*y=w241:dbl)
                        n135 = Index Array(array=w225, index (row)=w226) -> (element=w223:dbl[])  [unwired: 1 in]
                        n136 = Build Array(w261, w260, w251, w241, w234, w229, w207, w203) -> (w228:dbl[])
                        n137 = Array Subset(array=w223, index=8) -> (w222:dbl[])  [unwired: 1 in]
                        n138 = Build Array (concatenate)(w228, w222) -> (w227:dbl[])
                        n139 = Replace Array Subset(array=w225, new element=w227, index (row)=w226) -> (w224:dbl[][])  [unwired: 1 in]
                        n140 = local write "obs_tmp"(w224) -> ()
                      }
                      frame 1 {
                        w290 = u8 4 ("y")
                        n141 = Index Array(array=w305, index #1=0 ("index")) -> (element #1=w303:u8, element #2=w297:u8, element #3=w295:u8, element #4=w284:u8)  [unwired: 3 in]
                        n142 = local read "obs_tmp"() -> (w282:dbl[][])
                        n143 = And(x=w284, y=w290) -> (x .and. y?=w291:u8)
                        n144 = To Double Precision Float(number=w303) -> (double precision float=w302:dbl)
                        n145 = To Double Precision Float(number=w297) -> (double precision float=w298:dbl)
                        n146 = To Double Precision Float(number=w295) -> (double precision float=w294:dbl)
                        n147 = And(x=u8 3 ("y"), y=w284) -> (x .and. y?=w293:u8)
                        n148 = Equal?(x=w291, y=w290) -> (x = y?=w289:bool)
                        n149 = Index Array(array=w282, index (row)=w280) -> (element=w277:dbl[])  [unwired: 1 in]
                        n150 = To Double Precision Float(number=w293) -> (double precision float=w292:dbl)
                        n151 = Multiply(x=w302, y=0.5) -> (x*y=w300:dbl)
                        n152 = Multiply(x=w298, y=0.05) -> (x*y=w296:dbl)
                        n153 = Select(t=1.0, s=w289, f=0.0) -> (s? t:f=w286:dbl)
                        n154 = Array Subset(array=w277, index=13) -> (w273:dbl[])  [unwired: 1 in]
                        n155 = Build Array(w300, w296, w294, w292, w286) -> (w274:dbl[])
                        n156 = Array Subset(array=w277, index=0, length=8) -> (w275:dbl[])
                        n157 = Build Array (concatenate)(w275, w274, w273) -> (w283:dbl[])
                        n158 = Replace Array Subset(array=w282, new element=w283, index (row)=w280) -> (w281:dbl[][])  [unwired: 1 in]
                        n159 = local write "obs_tmp"(w281) -> ()
                      }
                      frame 2 {
                        n160 = flat-sequence {
                          tunnel: w308 -> [w359]
                          tunnel: w307 -> [w311]
                          tunnel: w306 -> [w310]
                          frame #0 {
                            w333 = i16 6 ("y")
                            n161 = Index Array(array=w359, index #1=1 ("index"), index #2=0 ("index"), index #3=3 ("index"), index #4=2 ("index"), index #5=5 ("index"), index #6=4 ("index"), index #7=7 ("index"), index #8=6 ("index")) -> (element #1=w356:u8, element #2=w355:u8, element #3=w343:u8, element #4=w342:u8, element #5=w338:u8, element #6=w337:u8, element #7=w321:u8, element #8=w320:u8)
                            n162 = Join Numbers(hi=w356, lo=w355) -> ((hi.lo)=w354:u16)
                            n163 = Join Numbers(hi=w343, lo=w342) -> ((hi.lo)=w344:u16)
                            n164 = Join Numbers(hi=w338, lo=w337) -> ((hi.lo)=w336:u16)
                            n165 = Join Numbers(hi=w321, lo=w320) -> ((hi.lo)=w322:u16)
                            n166 = Logical Shift(y=w333, x=w336) -> (x << y=w335:u16)
                            n167 = To Word Integer(number=w354) -> (16bit integer=w353:i16)
                            n168 = To Word Integer(number=w344) -> (16bit integer=w345:i16)
                            n169 = Negate(x=w333) -> (-x=w334:i16)
                            n170 = To Word Integer(number=w322) -> (16bit integer=w323:i16)
                            n171 = To Double Precision Float(number=w353) -> (double precision float=w352:dbl)
                            n172 = To Double Precision Float(number=w345) -> (double precision float=w346:dbl)
                            n173 = To Word Integer(number=w335) -> (16bit integer=w332:i16)
                            n174 = To Double Precision Float(number=w323) -> (double precision float=w324:dbl)
                            n175 = local read "obs_tmp"() -> (w318:dbl[][])
                            n176 = Scale By Power Of 2(n=w334, x=w332) -> (x*2^n=w331:i16)
                            n177 = Multiply(x=w352, y=0.01) -> (x*y=w350:dbl)
                            n178 = Multiply(x=w346, y=0.0002) -> (x*y=w341:dbl)
                            n179 = Index Array(array=w318, index (row)=w311) -> (element=w315:dbl[])  [unwired: 1 in]
                            n180 = To Double Precision Float(number=w331) -> (double precision float=w329:dbl)
                            n181 = Multiply(x=w324, y=0.01) -> (x*y=w319:dbl)
                            n182 = Array Subset(array=w315, index=0, length=13) -> (w312:dbl[])
                            n183 = Multiply(x=w329, y=0.03) -> (x*y=w328:dbl)
                            n184 = Build Array(w350, w341, w328, w319, w310) -> (w314:dbl[])
                            n185 = Build Array (concatenate)(w312, w314) -> (w313:dbl[])
                            n186 = Replace Array Subset(array=w318, new element=w313, index (row)=w311) -> (w309:dbl[][])  [unwired: 1 in]
                            n187 = global write "G_mobileye_Temp.vi" "obs"(w309) -> ()
                            n188 = local write "obs_tmp"(w309) -> ()
                          }
                        }
                      }
                    }
                  }
                }
              }
              frame 1898 {
                n189 = Index Array(array=w362, index=3) -> (element=w365:u8)
                n190 = Greater Or Equal?(x=w365, y=u8 128) -> (x >= y?=w363:bool)
                n191 = case shown="True" w363 {
                  tunnel: w362 -> [_ w392]
                  tunnel: [_ w367] -> w361
                  tunnel: [_ w369] -> w360
                  frame False {
                  }
                  frame True {
                    n192 = Index Array(array=w392, index #1=3 ("index"), index #2=2 ("index"), index #3=1 ("index"), index #4=0 ("index")) -> (element #1=w383:u8, element #2=w387:u8, element #3=w386:u8, element #4=w385:u8)
                    n193 = Join Numbers(hi=w386, lo=w385) -> ((hi.lo)=w373:u16)
                    n194 = Subtract(x=w383, y=u8 128) -> (x-y=w382:u8)
                    n195 = Join Numbers(hi=w382, lo=w387) -> ((hi.lo)=w375:u16)
                    n196 = To Double Precision Float(number=w373) -> (double precision float=w381:dbl)
                    n197 = To Double Precision Float(number=u16 2047 ("(hi.lo)")) -> (double precision float=w380:dbl)
                    n198 = Subtract(x=w381, y=w380) -> (x-y=w378:dbl)
                    n199 = To Double Precision Float(number=w375) -> (double precision float=w374:dbl)
                    n200 = Divide(x=w374, y=256.0) -> (x/y=w372:dbl)
                    n201 = Divide(x=w378, y=256.0) -> (x/y=w369:dbl)
                    n202 = Square(x=w372) -> (x^2=w371:dbl)
                    n203 = Square(x=w369) -> (x^2=w370:dbl)
                    n204 = Subtract(x=w371, y=w370) -> (x-y=w368:dbl)
                    n205 = Square Root(x=w368) -> (sqrt(x)=w367:dbl)
                  }
                }
                n206 = Build Array(w361, w360) -> ()  [unwired: 1 out]
              }
              frame 1894, 1896, 1900, 1902, 1904, 1906, 1908, 1910, 1912, 1914 {
                n207 = Index Array(array=w447, index #1=0 ("index"), index #2=7 ("index"), index #3=2 ("index"), index #4=1 ("index"), index #5=4 ("index"), index #6=3 ("index"), index #7=6 ("index"), index #8=5 ("index")) -> (element #1=w403:u8, element #2=w398:u8, element #3=w445:u8, element #4=w444:u8, element #5=w437:u8, element #6=w436:u8, element #7=w427:u8, element #8=w426:u8)
                n208 = Join Numbers(hi=w445, lo=w444) -> ((hi.lo)=w443:u16)
                n209 = Join Numbers(hi=w437, lo=w436) -> ((hi.lo)=w435:u16)
                n210 = Join Numbers(hi=w427, lo=w426) -> ((hi.lo)=w420:u16)
                n211 = And(x=w403, y=u8 48) -> (x .and. y?=w408:u8)
                n212 = To Word Integer(number=w443) -> (16bit integer=w442:i16)
                n213 = To Double Precision Float(number=w435) -> (double precision float=w432:dbl)
                n214 = To Double Precision Float(number=w420) -> (double precision float=w423:dbl)
                n215 = Logical Shift(y=i16 -4, x=w408) -> (x << y=w406:u8)
                n216 = To Double Precision Float(number=u16 32767 ("y")) -> (double precision float=w433:dbl)
                n217 = To Double Precision Float(number=u16 32767 ("y")) -> (double precision float=w422:dbl)
                n218 = Logical Shift(y=28, x=1) -> (x << y=w417:i32)
                n219 = Subtract(x=w432, y=w433) -> (x-y=w431:dbl)
                n220 = Subtract(x=w423, y=w422) -> (x-y=w415:dbl)
                n221 = To Double Precision Float(number=w417) -> (double precision float=w416:dbl)
                n222 = Logical Shift(y=i16 -6, x=w403) -> (x << y=w401:u8)
                n223 = Divide(x=w442, y=i16 256) -> (x/y=w428:dbl)
                n224 = Divide(x=w415, y=w416) -> (x/y=w414:dbl)
                n225 = To Double Precision Float(number=w406) -> (double precision float=w404:dbl)
                n226 = And(x=u8 15, y=w403) -> (x .and. y?=w410:u8)
                n227 = Multiply(x=w398, y=0.01) -> (x*y=w396:dbl)
                n228 = Divide(x=w431, y=1024000.0) -> (x/y=w429:dbl)
                n229 = To Double Precision Float(number=w413) -> (double precision float=w395:dbl)
                n230 = To Double Precision Float(number=w410) -> (double precision float=w405:dbl)
                n231 = To Double Precision Float(number=w401) -> (double precision float=w400:dbl)
                n232 = Build Array(w395, w405, w404, w400, w396, w428, w429, w414) -> (w394:dbl[])
                n233 = case shown="76C, 770, 774, 778" w393 {
                  selector: w393 -> [_ _ _ w463 w471]
                  tunnel: w394 -> [_ w449 w455 w464 w472]
                  frame 0, Default {
                  }
                  frame 1894 {
                    n234 = local read "lane_left"() -> (w452:dbl[])
                    n235 = Array Subset(array=w452, index=8) -> (w450:dbl[])  [unwired: 1 in]
                    n236 = Build Array (concatenate)(w449, w450) -> (w448:dbl[])
                    n237 = local write "lane_left"(w448) -> ()
                  }
                  frame 1896 {
                    n238 = local read "lane_right"() -> (w457:dbl[])
                    n239 = Array Subset(array=w457, index=8) -> (w454:dbl[])  [unwired: 1 in]
                    n240 = Build Array (concatenate)(w455, w454) -> (w453:dbl[])
                    n241 = local write "lane_right"(w453) -> ()
                  }
                  frame 1900, 1904, 1908, 1912 {
                    n242 = Subtract(x=w463, y=u32 1900) -> (x-y=w461:u32)
                    n243 = Quotient & Remainder(x=w461, y=u32 4) -> (floor(x/y)=w459:u32)  [unwired: 1 out]
                    n244 = local read "next lane left"() -> (w465:dbl[][])
                    n245 = Replace Array Subset(array=w465, new element=w464, index (row)=w459) -> (w458:dbl[][])  [unwired: 1 in]
                    n246 = local write "next lane left"(w458) -> ()
                  }
                  frame 1902, 1906, 1910, 1914 {
                    n247 = Subtract(x=w471, y=u32 1900) -> (x-y=w469:u32)
                    n248 = local read "next lane right"() -> (w473:dbl[][])
                    n249 = Quotient & Remainder(x=w469, y=u32 4) -> (floor(x/y)=w467:u32)  [unwired: 1 out]
                    n250 = Replace Array Subset(array=w473, new element=w472, index (row)=w467) -> (w466:dbl[][])  [unwired: 1 in]
                    n251 = local write "next lane right"(w466) -> ()
                  }
                }
              }
              frame 1895, 1897, 1901, 1903, 1905, 1907, 1909, 1911, 1913, 1915 {
                w485 = u16 32768 ("y")
                n252 = Index Array(array=w502, index #1=1 ("index"), index #2=0 ("index"), index #3=3 ("index"), index #4=2 ("index")) -> (element #1=w499:u8, element #2=w498:u8, element #3=w489:u8, element #4=w488:u8)
                n253 = Join Numbers(hi=w499, lo=w498) -> ((hi.lo)=w494:u16)
                n254 = Join Numbers(hi=w489, lo=w488) -> ((hi.lo)=w486:u16)
                n255 = Subtract(x=w486, y=w485) -> (x-y=w484:u16)
                n256 = And(x=w485, y=w486) -> (x .and. y?=w487:u16)
                n257 = To Double Precision Float(number=w494) -> (double precision float=w495:dbl)
                n258 = To Double Precision Float(number=u16 32767 ("y")) -> (double precision float=w496:dbl)
                n259 = Equal?(x=w485, y=w487) -> ()  [unwired: 1 out]
                n260 = Subtract(x=w495, y=w496) -> (x-y=w493:dbl)
                n261 = Divide(x=w484, y=u16 256) -> (x/y=w482:dbl)
                n262 = Select(t=w482, s=TRUE, f=0.0) -> (s? t:f=w479:dbl)
                n263 = Divide(x=w493, y=1024.0) -> (x/y=w480:dbl)
                n264 = To Double Precision Float(number=w478) -> (double precision float=w477:dbl)
                n265 = Build Array(w477, w480, w479) -> (w476:dbl[])
                n266 = case shown="76D, 771, 775, 779" w475 {
                  selector: w475 -> [_ _ _ w524 w539]
                  tunnel: w476 -> [_ w504 w510 w520 w535]
                  frame 0, Default {
                  }
                  frame 1895 {
                    n267 = local read "lane_left"() -> (w508:dbl[])
                    n268 = Array Subset(array=w508, index=0, length=8 ("index")) -> (w507:dbl[])
                    n269 = Build Array (concatenate)(w507, w504) -> (w503:dbl[])
                    n270 = local write "lane_left"(w503) -> ()
                    n271 = global write "G_mobileye_Temp.vi" "lane_left"(w503) -> ()
                  }
                  frame 1897 {
                    n272 = local read "lane_right"() -> (w514:dbl[])
                    n273 = Array Subset(array=w514, index=0, length=8 ("index")) -> (w513:dbl[])
                    n274 = Build Array (concatenate)(w513, w510) -> (w509:dbl[])
                    n275 = local write "lane_right"(w509) -> ()
                    n276 = global write "G_mobileye_Temp.vi" "lane_right"(w509) -> ()
                  }
                  frame 1901, 1905, 1909, 1913 {
                    n277 = Subtract(x=w524, y=u32 1900) -> (x-y=w527:u32)
                    n278 = local read "next lane left"() -> (w529:dbl[][])
                    n279 = Quotient & Remainder(x=w527, y=u32 4) -> (floor(x/y)=w521:u32)  [unwired: 1 out]
                    n280 = Index Array(array=w520, index #1=0 ("index")) -> (element #1=w518:dbl, element #2=w517:dbl, element #3=w516:dbl)  [unwired: 2 in]
                    n281 = Replace Array Subset(array=w529, new element #1=w518, index (row) #1=w521, index (col) #1=8 ("disabled index (col)"), new element #2=w517, index (row) #2=w521, index (col) #2=9 ("disabled index (col)"), new element #3=w516, index (row) #3=w521, index (col) #3=10 ("index (col)")) -> (w515:dbl[][])
                    n282 = local write "next lane left"(w515) -> ()
                    n283 = global write "G_mobileye_Temp.vi" "lane_left 2"(w515) -> ()
                  }
                  frame 1903, 1907, 1911, 1915 {
                    n284 = Subtract(x=w539, y=u32 1900) -> (x-y=w542:u32)
                    n285 = local read "next lane right"() -> (w544:dbl[][])
                    n286 = Quotient & Remainder(x=w542, y=u32 4) -> (floor(x/y)=w536:u32)  [unwired: 1 out]
                    n287 = Index Array(array=w535, index #1=0 ("index")) -> (element #1=w533:dbl, element #2=w532:dbl, element #3=w531:dbl)  [unwired: 2 in]
                    n288 = Replace Array Subset(array=w544, new element #1=w533, index (row) #1=w536, index (col) #1=8 ("disabled index (col)"), new element #2=w532, index (row) #2=w536, index (col) #2=9 ("disabled index (col)"), new element #3=w531, index (row) #3=w536, index (col) #3=10 ("index (col)")) -> (w530:dbl[][])
                    n289 = local write "next lane right"(w530) -> ()
                    n290 = global write "G_mobileye_Temp.vi" "lane_right 2"(w530) -> ()
                  }
                }
              }
            }
          }
        }
      }
    }
  }
  n291 = disable-structure shown="Enabled" {
    frame Enabled {
      n292 = while {
        stop <- FALSE stop-if-true
        n293 = flat-sequence {
          tunnel: [w608] -> w551
          tunnel: [w607] -> w550
          tunnel: [w606] -> w548
          tunnel: [w605] -> w545
          tunnel: [w714] -> w554
          tunnel: [w713] -> w553
          tunnel: [w712] -> w552
          tunnel: w551 -> [w712]
          tunnel: w550 -> [w711]
          tunnel: [w711] -> w549
          tunnel: w548 -> [w710]
          tunnel: [w710] -> w547
          tunnel: [w709] -> w546
          tunnel: w545 -> [w709]
          tunnel: w554 -> [w766]
          tunnel: w553 -> [w767]
          tunnel: w552 -> [w771]
          tunnel: w549 -> [w770]
          tunnel: w547 -> [w769]
          tunnel: w546 -> [w768]
          frame #0 {
            n294 = Wait Until Next ms Multiple(millisecond multiple=u32 10) -> ()  [unwired: 1 out]
          }
          frame #1 {
            n295 = global read "G_mobileye_Temp.vi" "lane_right"() -> (w563:dbl[])
            n296 = global read "G_mobileye_Temp.vi" "lane_left"() -> (w564:dbl[])
            n297 = Index Array(array=w564, index=10) -> (element=w566:dbl)
            n298 = Index Array(array=w563, index=10) -> (element=w575:dbl)
            n299 = Multiply(x=w566, y=2.0) -> (x*y=w567:dbl)
            n300 = Multiply(x=w575, y=2.0) -> (x*y=w574:dbl)
            n301 = Round Toward -Infinity(1:w567) -> (0:w558:dbl)
            n302 = Round Toward -Infinity(1:w574) -> (0:w562:dbl)
            n303 = Max & Min(x=10.0, y=w558) -> (max(x,y)=w557:dbl)  [unwired: 1 out]
            n304 = Max & Min(x=10.0, y=w562) -> (max(x,y)=w560:dbl)  [unwired: 1 out]
            n305 = local read "x_view"() -> (w568:dbl[])
            n306 = local read "x_view"() -> (w573:dbl[])
            n307 = Array Subset(array=w568, index=0, length=w557) -> (w577:dbl[])
            n308 = Array Subset(array=w573, index=0, length=w560) -> (w578:dbl[])
            n309 = global write "G_mobileye_Temp.vi" "x_l"(w577) -> ()
            n310 = global write "G_mobileye_Temp.vi" "x_r"(w578) -> ()
            n311 = Index Array(array=w564, index #1=7 ("index"), index #2=6 ("index"), index #3=9 ("index"), index #4=5 ("index")) -> (element #1=w582:dbl, element #2=w584:dbl, element #3=w586:dbl, element #4=w590:dbl)
            n312 = Index Array(array=w563, index #1=7 ("index"), index #2=6 ("index"), index #3=9 ("index"), index #4=5 ("index")) -> (element #1=w603:dbl, element #2=w601:dbl, element #3=w599:dbl, element #4=w595:dbl)
            n313 = Square(x=w577) -> (x^2=w580:dbl[])
            n314 = Square(x=w578) -> (x^2=w579:dbl[])
            n315 = Compound Arithmetic op=MULTIPLY(w582, w577, w580) -> (w587:dbl[])
            n316 = Compound Arithmetic op=MULTIPLY(w580, w584) -> (w588:dbl[])
            n317 = Compound Arithmetic op=MULTIPLY(w577, w586) -> (w589:dbl[])
            n318 = Compound Arithmetic op=MULTIPLY(w603, w578, w579) -> (w598:dbl[])
            n319 = Compound Arithmetic op=MULTIPLY(w579, w601) -> (w597:dbl[])
            n320 = Compound Arithmetic op=MULTIPLY(w578, w599) -> (w596:dbl[])
            n321 = Compound Arithmetic op=ADD(w587, w588, w589, w590) -> (w592:dbl[])
            n322 = Compound Arithmetic op=ADD(w598, w597, w596, w595) -> (w593:dbl[])
            n323 = global write "G_mobileye_Temp.vi" "y_l"(w592) -> ()
            n324 = global write "G_mobileye_Temp.vi" "y_r"(w593) -> ()
          }
          frame #2 {
            n325 = disable-structure shown="Enabled" {
              disable-tunnel: [w630 _] -> w608
              disable-tunnel: [w629 _] -> w607
              disable-tunnel: [w616 _] -> w606
              disable-tunnel: [w615 _] -> w605
              frame Enabled {
                w628 = dynamicdata [] ("Dynamic Data Type")
                w631 = dynamicdata [] ("Dynamic Data Type")
                n326 = global read "G_mobileye_Temp.vi" "lane_right 2"() -> (w632:dbl[][])
                n327 = global read "G_mobileye_Temp.vi" "lane_left 2"() -> (w627:dbl[][])
                n328 = global read "G_mobileye_Temp.vi" "mobileye time"() -> (w634:u32)
                n329 = global read "G_mobileye_Temp.vi" "mobileye time"() -> (w625:u32)
                n330 = Index Array(array=w632, index (col)=0 ("disabled index (col)")) -> (element=w633:dbl[])  [unwired: 1 in]
                n331 = Index Array(array=w627, index (col)=0 ("disabled index (col)")) -> (element=w626:dbl[])  [unwired: 1 in]
                n332 = Subtract(x=w633, y=w634) -> (x-y=w635:dbl[])
                n333 = Subtract(x=w626, y=w625) -> (x-y=w624:dbl[])
                n334 = Multiply(x=w635, y=1e-06) -> (x*y=w637:dbl[])
                n335 = Multiply(x=w624, y=1e-06) -> (x*y=w622:dbl[])
                n336 = Absolute Value(x=w637) -> (abs(x)=w638:dbl[])
                n337 = Absolute Value(x=w622) -> (abs(x)=w621:dbl[])
                n338 = Less?(x=w638, y=1.0) -> (x < y?=w640:bool[])
                n339 = Less?(x=w621, y=1.0) -> (x < y?=w619:bool[])
                n340 = Boolean To (0,1)(Boolean=w640) -> (0, 1=w641:i16[])
                n341 = Boolean To (0,1)(Boolean=w619) -> (0, 1=w618:i16[])
                n342 = Add Array Elements(numeric array=w641) -> (sum=w614:i16)
                n343 = Add Array Elements(numeric array=w618) -> (sum=w610:i16)
                n344 = Max & Min(x=i16 1, y=w614) -> (min(x,y)=w613:i16)  [unwired: 1 out]
                n345 = Max & Min(x=i16 1, y=w610) -> (min(x,y)=w609:i16)  [unwired: 1 out]
                n346 = for {
                  N: w613 -> [_]
                  tunnel: w632 -> [w676] mode=indexing
                  shift-right: [w685] -> w629
                  shift-left: w631 -> [w686]
                  shift-right: [w681] -> w630
                  shift-left: w631 -> [w682]
                  n347 = disable-structure shown="Enabled" {
                    disable-tunnel: [w707 w708] -> w680
                    disable-tunnel: w676 -> [_ w708]
                    frame Disabled {
                      n348 = global read "G_mobileye_Temp.vi" "lane_right"() -> (w707:dbl[])
                    }
                    frame Enabled {
                    }
                  }
                  n349 = Index Array(array=w676, index=5) -> (element=w678:dbl)
                  n350 = Index Array(array=w680, index=10) -> (element=w700:dbl)
                  n351 = Multiply(x=w700, y=1.8) -> (x*y=w677:dbl)
                  n352 = Round Toward -Infinity(1:w677) -> (0:w704:dbl)
                  n353 = Max & Min(x=5.0, y=w704) -> (max(x,y)=w706:dbl)  [unwired: 1 out]
                  n354 = local read "x_view"() -> (w701:dbl[])
                  n355 = Index Array(array=w680, index #1=7 ("index"), index #2=6 ("index"), index #3=9 ("index")) -> (element #1=w690:dbl, element #2=w692:dbl, element #3=w694:dbl)
                  n356 = Array Subset(array=w701, index=0, length=w706) -> (w688:dbl[])
                  n357 = Square(x=w688) -> (x^2=w698:dbl[])
                  n358 = call "Convert to Dynamic Data7"("Array"=w688) -> ("Dynamic Data Type"=w687:dynamicdata)  [unwired: 3 in]
                  n359 = Compound Arithmetic op=MULTIPLY(w688, w694) -> (w697:dbl[])
                  n360 = Merge Signals(w686, w687) -> (w685:dynamicdata)
                  n361 = Compound Arithmetic op=MULTIPLY(w690, w688, w698) -> (w695:dbl[])
                  n362 = Compound Arithmetic op=MULTIPLY(w698, w692) -> (w696:dbl[])
                  n363 = Compound Arithmetic op=ADD(w695, w696, w697, w678) -> (w683:dbl[])
                  n364 = call "Convert to Dynamic Data8"("Array"=w683) -> ("Dynamic Data Type"=w684:dynamicdata)  [unwired: 3 in]
                  n365 = Merge Signals(w682, w684) -> (w681:dynamicdata)
                }
                n366 = for {
                  N: w609 -> [_]
                  tunnel: w627 -> [w643] mode=indexing
                  shift-right: [w651] -> w615
                  shift-left: w628 -> [w652]
                  shift-right: [w647] -> w616
                  shift-left: w628 -> [w648]
                  n367 = disable-structure shown="Enabled" {
                    disable-tunnel: [w674 w675] -> w646
                    disable-tunnel: w643 -> [_ w675]
                    frame Disabled {
                      n368 = global read "G_mobileye_Temp.vi" "lane_left"() -> (w674:dbl[])
                    }
                    frame Enabled {
                    }
                  }
                  n369 = Index Array(array=w643, index=5) -> (element=w644:dbl)
                  n370 = Index Array(array=w646, index=10) -> (element=w666:dbl)
                  n371 = Multiply(x=w666, y=1.8) -> (x*y=w667:dbl)
                  n372 = Round Toward -Infinity(1:w667) -> (0:w671:dbl)
                  n373 = Max & Min(x=5.0, y=w671) -> (max(x,y)=w673:dbl)  [unwired: 1 out]
                  n374 = local read "x_view"() -> (w668:dbl[])
                  n375 = Index Array(array=w646, index #1=7 ("index"), index #2=6 ("index"), index #3=9 ("index")) -> (element #1=w656:dbl, element #2=w658:dbl, element #3=w660:dbl)
                  n376 = Array Subset(array=w668, index=0, length=w673) -> (w654:dbl[])
                  n377 = Square(x=w654) -> (x^2=w664:dbl[])
                  n378 = call "Convert to Dynamic Data11"("Array"=w654) -> ("Dynamic Data Type"=w653:dynamicdata)  [unwired: 3 in]
                  n379 = Compound Arithmetic op=MULTIPLY(w654, w660) -> (w663:dbl[])
                  n380 = Merge Signals(w652, w653) -> (w651:dynamicdata)
                  n381 = Compound Arithmetic op=MULTIPLY(w656, w654, w664) -> (w661:dbl[])
                  n382 = Compound Arithmetic op=MULTIPLY(w664, w658) -> (w662:dbl[])
                  n383 = Compound Arithmetic op=ADD(w661, w662, w663, w644) -> (w649:dbl[])
                  n384 = call "Convert to Dynamic Data12"("Array"=w649) -> ("Dynamic Data Type"=w650:dynamicdata)  [unwired: 3 in]
                  n385 = Merge Signals(w648, w650) -> (w647:dynamicdata)
                }
              }
              frame Disabled {
              }
            }
          }
          frame #3 {
            w718 = dynamicdata [] ("Dynamic Data Type")
            n386 = global read "G_mobileye_Temp.vi" "obs"() -> (w717:dbl[][])
            n387 = global read "G_mobileye_Temp.vi" "mobileye time"() -> (w716:u32)
            n388 = Index Array(array=w717, index (col)=17 ("disabled index (col)")) -> (element=w726:dbl[])  [unwired: 1 in]
            n389 = Subtract(x=w726, y=w716) -> (x-y=w725:dbl[])
            n390 = Multiply(x=w725, y=1e-06) -> (x*y=w723:dbl[])
            n391 = Absolute Value(x=w723) -> (abs(x)=w722:dbl[])
            n392 = Less?(x=w722, y=1.0) -> (x < y?=w720:bool[])
            n393 = Boolean To (0,1)(Boolean=w720) -> (0, 1=w719:i16[])
            n394 = Add Array Elements(numeric array=w719) -> (sum=w715:i16)
            n395 = for {
              N: w715 -> [_]
              tunnel: w717 -> [w762] mode=indexing
              shift-right: [w744] -> w714
              shift-left: w718 -> [w746]
              shift-right: [w742] -> w713
              shift-left: w718 -> [w741]
              w732 = 0.0 ("element")
              w748 = 0.0 ("x0")
              n396 = Index Array(array=w762, index #1=2 ("index"), index #2=8 ("index"), index #3=9 ("index"), index #4=16 ("index"), index #5=1 ("index")) -> (element #1=w736:dbl, element #2=w731:dbl, element #3=w759:dbl, element #4=w754:dbl, element #5=w737:dbl)
              n397 = Max & Min(x=w731, y=5.0) -> (min(x,y)=w729:dbl)  [unwired: 1 out]
              n398 = Multiply(x=w754, y=3.141592653589793) -> (x*y=w752:dbl)
              n399 = Multiply(x=w759, y=0.5) -> (x*y=w757:dbl)
              n400 = Negate(x=w757) -> (-x=w756:dbl)
              n401 = Divide(x=w752, y=180.0) -> (x/y=w747:dbl)
              n402 = Build Array(w756, w757, w757, w756, w756) -> (w750:dbl[])
              n403 = Build Array(w732, w732, w729, w729, w732) -> (w749:dbl[])
              n404 = Negate(x=w736) -> (-x=w735:dbl)
              n405 = call "rotm_obs_new.vi"("angle[rad]"=w747, "y0"=w748, "x0"=w748, "y"=w749, "x"=w750) -> ("rot*(y-y0) 2"=w740:dbl[], "rot*(x-x0)"=w734:dbl[])  [unwired: 3 in, 2 out]
              n406 = Add(x=w735, y=w734) -> (x+y=w733:dbl[])
              n407 = Add(x=w740, y=w737) -> (x+y=w739:dbl[])
              n408 = call "Convert to Dynamic Data9"("Array"=w733) -> ("Dynamic Data Type"=w745:dynamicdata)  [unwired: 3 in]
              n409 = call "Convert to Dynamic Data10"("Array"=w739) -> ("Dynamic Data Type"=w743:dynamicdata)  [unwired: 3 in]
              n410 = Merge Signals(w746, w745) -> (w744:dynamicdata)
              n411 = Merge Signals(w741, w743) -> (w742:dynamicdata)
            }
          }
          frame #4 {
            n412 = global read "G_mobileye_Temp.vi" "y_r"() -> (w782:dbl[])
            n413 = global read "G_mobileye_Temp.vi" "y_l"() -> (w780:dbl[])
            n414 = global read "G_mobileye_Temp.vi" "x_r"() -> (w781:dbl[])
            n415 = call "Convert to Dynamic Data"("Array"=w782) -> ("Dynamic Data Type"=w785:dynamicdata)  [unwired: 3 in]
            n416 = call "Convert to Dynamic Data3"("Array"=w780) -> ("Dynamic Data Type"=w779:dynamicdata)  [unwired: 3 in]
            n417 = call "Convert to Dynamic Data5"("Array"=dbl[] [-0.94, 0.94, 0.94, -0.94, -0.94] ("appended array 2")) -> ("Dynamic Data Type"=w773:dynamicdata)  [unwired: 3 in]
            n418 = Add(x=dbl[] [-3.5, -3.5, 1.2, 1.2, -3.5] ("appended array"), y=0.3) -> (x+y=w764:dbl[])
            n419 = global read "G_mobileye_Temp.vi" "x_l"() -> (w777:dbl[])
            n420 = Merge Signals(w785, w779, w773, w771, w769, w766) -> (w775:dynamicdata)
            n421 = call "Convert to Dynamic Data2"("Array"=w781) -> ("Dynamic Data Type"=w784:dynamicdata)  [unwired: 3 in]
            n422 = call "Convert to Dynamic Data6"("Array"=w764) -> ("Dynamic Data Type"=w772:dynamicdata)  [unwired: 3 in]
            n423 = call "Convert to Dynamic Data4"("Array"=w777) -> ("Dynamic Data Type"=w776:dynamicdata)  [unwired: 3 in]
            n424 = Merge Signals(w784, w776, w772, w770, w768, w767) -> (w778:dynamicdata)
            n425 = call "Build XY Graph"("Y Input"=w778, "X Input"=w775) -> ("XY Graph"=→"XY Graph":cluster{"X":dbl[], "Y":dbl[]}[])  [unwired: 8 in, 1 out]
          }
        }
      }
    }
    frame Disabled {
    }
  }
  n426 = while {
    stop <- FALSE stop-if-true
    n427 = global read "G_LCM.vi" "CAN_CAR_RAW_T"() -> (w787:T3)
    n428 = Unbundle By Name(w787) -> ("car time"=w789:u32)
    n429 = feedback-in #2(w789) -> ()
    n430 = feedback #2(u32 0 ("mobileye time")) -> (w790:u32)
    n431 = Not Equal?(x=w789, y=w790) -> (x != y?=w788:bool)
    n432 = case shown="True" w788 {
      tunnel: w787 -> [_ w799]
      frame False {
      }
      frame True {
        n433 = Unbundle By Name(w799) -> ("ID"=w798:u32, "data"=w797:u8[], "car time"=w793:u32)
        n434 = Multiply(x=w793, y=1e-07) -> (x*y=w792:dbl)
        n435 = To Time Stamp(1:w792) -> (0:w796:timestamp)
        n436 = Bundle By Name(cluster=T2 {"identifier"=0, "timestamp"=timestamp(0 s since 1904-01-01), "payload"=[]} ("can cluster"), "identifier"=w798, "payload"=w797, "timestamp"=w796) -> (w800:T2)
        n437 = call "can decoder.vi"("can cluster"=w800, "name"="Avante") -> ()  [unwired: 10 in]
      }
    }
  }
